vi "Dashboard Main.vi"() -> ()   [LabVIEW 2013]
uses:
  <vilib>/event_ctls.llb/eventvkey.ctl
  <vilib>/Rock Robotics/WPI/Dashboard/WPI_DashboardLogging Global.vi
  <vilib>/Utility/config.llb/Write Key (String).vi
  <vilib>/Utility/config.llb/Write Key (I32).vi
  <vilib>/Utility/config.llb/NI_LVConfig.lvlib
panel:
  out "LED 1":bool
  out "MotorSlide4 2":dbl(slide) scale=0.0..14.0 scale format="%#_2e"
  out "MotorSlide2 2":dbl(slide) scale=-1.0..1.0 scale format="%#_2e"
  out "MotorSlide1 2":dbl(slide) scale=-1.0..1.0 scale format="%#_2e"
  out "MotorSlide2":dbl(slide) scale=-1.0..1.0 scale format="%#_2e"
  out "MotorSlide1":dbl(slide) scale=-1.0..1.0 scale format="%#_2e"
  out "JS1 Z":dbl(slide) scale=-1.0..1.0 scale format="%#_2e"
  out "Joystick 1":cluster{"X":dbl, "Y":dbl}[](graph)
  out "JS Buttons 1":T1
  out "JS2 Z":dbl(slide) scale=-1.0..1.0 scale format="%#_2e"
  out "Joystick 2":cluster{"X":dbl, "Y":dbl}[](graph)
  out "JS Buttons 2":T1
  out "MotorChart R":cluster{"Numeric":dbl, "Numeric":dbl}(graph)
  out "MotorChart L":T2(graph)
  in  "DB Camera Config":bool
  out "fps":dbl format="%#.1g"
  out "Mbps":dbl format="%#.1g"
  out "Mbps 2":bool
  out "Image Message":string="Timeout in Camera Communications"
  in  "Rec Mode":enum32{"Stop", "Record", "Playback"}(radio)
  in  "Dashboard Tab":T3(tab)
  out "Posicionado?":bool
  out "Distância":dbl(slide)=60.0 scale=0.0..140.0 scale format="%#.3g"
  out "MARCHA":string
  out "Tração Invertida":bool
  out "Bola Coletada?":bool
  out "Engatilhado?":bool
  out "Claw Open?":bool
  out "Arm Down?":bool
  out "Shooter angle ready?":bool
  in  "Camera Settings":T4={"Frame Rate"=30, "Compression"=30, "Size"=1} {"Frame Rate" scale=1.0..30.0; "Size" items=["640x480", "320x240", "160x120"]}
  out "Mode":T5(ring)=enum."Auto Disabled"
  out "Camera IP":string
  in  "Checkbox 2":bool
  in  "Checkbox 1":bool
  in  "Test Slider":dbl(slide) scale=0.0..100.0 scale format="%#_3g"
  in  "On/Off":bool caption="Solenoid"
  in  "Test Name":u16(ring) items=["Select the test to run...", "Example Test", "-------------------------------", "List of tests is built in robot code.", "Replace with your own automated tests."]
  in  "Test Tree":string(tree)
  in  "Motor":cluster{"Value":dbl, "Enable":bool} {"Value" scale=-1.0..1.0 scale format="%#_3g"}
  out "Progress":T6 {"Test Progress" scale=0.0..100.0}
  in  "Rev/Fwd":cluster{"Forward":bool, "Reverse":bool}
  in  "Test Ring":u16(ring) items=["Auto", "Fixed indoor", "Fixed outdoor 1", "Fixed outdoor 2", "Fixed fluorescent 1", "Fixed fluorescent 2", "Hold current"]
  in  "Listbox":i32(listbox)
  out "Tree":string(tree)
  out "Camera Image":T7(plugin-control)
  in  "Enable":bool
  # "ABRIR\nGARRA"
  # "PARA"
  # "REVERTE"
  # "INTAKE"
  # "BRAÇO"
  # "SHOOT GOAL"
  # "SOLTA\nSHOOTER"
  # "SHOOT\nTRUSS"
  # "Left"
  # "Right"
  # "Front"
  # "Battery"
  # "Movimento Da Garra"
  # "Ações Da Garra"
  # "Tração"
  # "This tab is a great place for autonomous settings and validation.\nCustomize by placing controls and indicators here and name to\nmatch Dashboard Variables on robot."
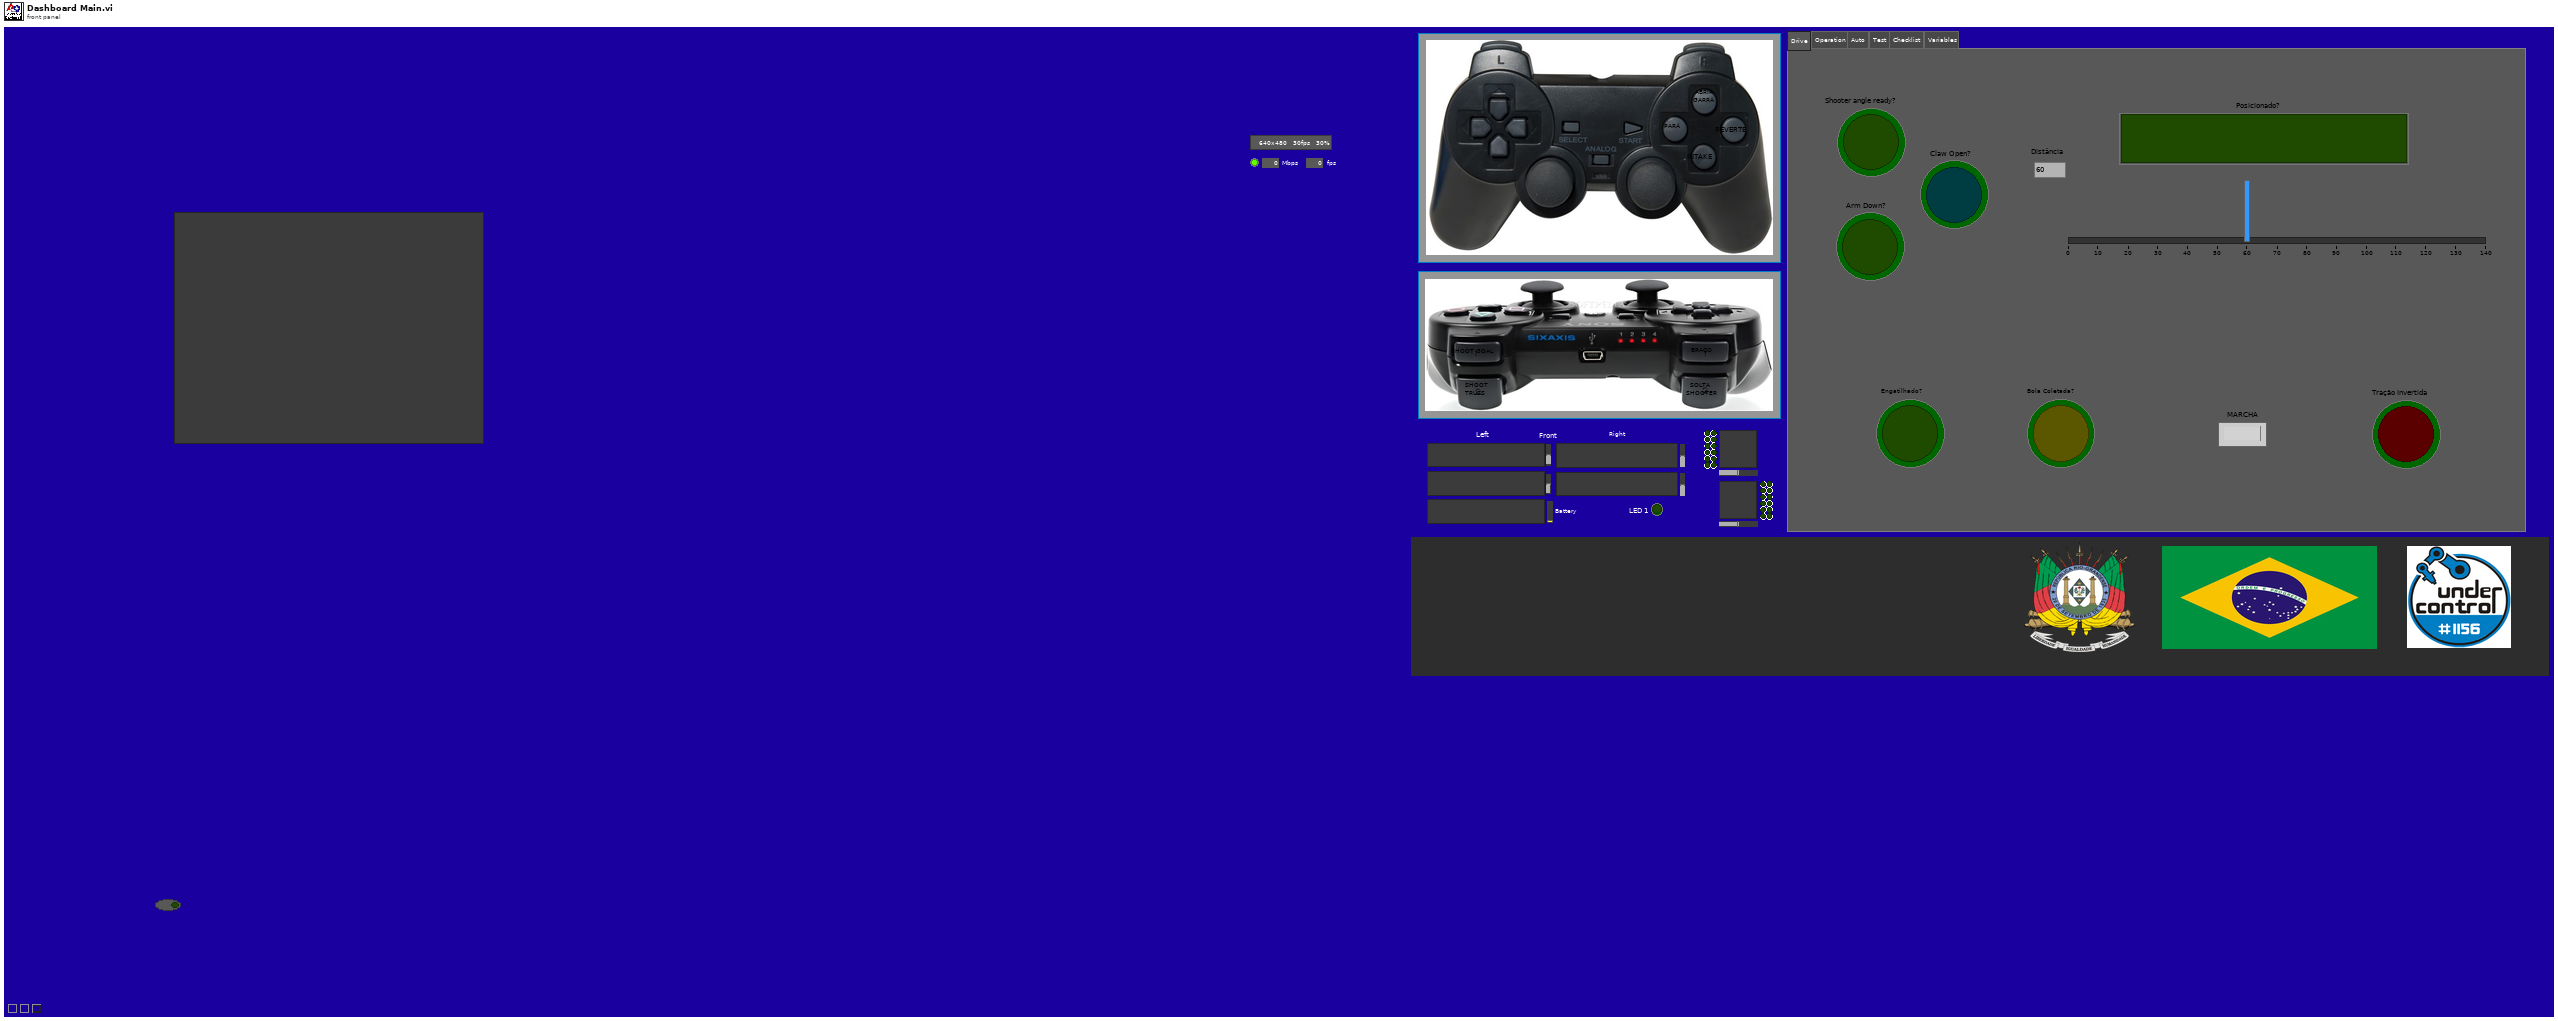
[diagram p1: front panel]
types:
  T1 = cluster{bool, bool, bool, bool, bool, bool, bool, bool, bool, bool, bool, bool}
  T2 = cluster{"Numeric":dbl, "Numeric":dbl, "Battery":sgl}
  T3 = enum32{"Drive", "Operation", "Auto", "Test", "Checklist", "Variables"}
  T4 = cluster{"Frame Rate":i32, "Compression":i32, "Size":u16}
  T5 = enum8{"Tele-Op Disabled", "Tele-Op Enabled", "Auto Disabled", "Auto Enabled", "Test Disabled", "Test Enabled", ""}
  T6 = cluster{"Test Progress":u8, "Test Progress Text":string}
  T7 = typedef "IMAQ Image.ctl" = refnum<image>
  T8 = typedef "Image Type" = u32
  T9 = cluster{"Digital Inputs":bool[], "Digital Outputs":bool[]}
  T10 = cluster{"Competition mode":bool, "Robot Link":bool, "Autonomous":bool, "Enabled":bool, "E-Stop":bool, "Simulated":bool, "TestMode":bool, "Docked Window":bool}
  T11 = cluster{"Boolean Array[0]":bool, "Boolean Array[1]":bool, "Boolean Array[2]":bool, "Boolean Array[3]":bool, "Boolean Array[4]":bool, "Boolean Array[5]":bool, "Boolean Array[6]":bool, "Boolean Array[7]":bool, "Boolean Array[8]":bool, "Boolean Array[9]":bool, "Boolean Array[10]":bool, "Boolean Array[11]":bool}
  T12 = typedef "NI_LVConfig.lvlib/Config Data RefNum.ctl" = refnum<k1>
  T13 = typedef "eventvkey.ctl" = enum16{"ASCII", "Enter", "Return", "Shift", "Ctrl", "Alt", "Cmd", "Opt", "Caps", "NumLock", "Clear", "Break", "Up", "Down", "Left", "Right", "Insert", "Delete", "Home", "End", "PageUp", "PageDown", "Escape", "Help", "Pause", "ScrollLock", "F1", "F2", "F3", "F4", "F5", "F6", "F7", "F8", "F9", "F10", "F11", "F12", "F13", "F14", "F15", "F16", "F17", "F18", "F19", "F20", "F21", "F22", "F23", "F24", "Play", "VolumeUp", "VolumeDown", "Mute", "Two Byte Char"}
  T14 = cluster{"Image Size":bool, "Image Type":bool, "Pixel Value":bool, "ROI Information":bool, "Zoom Factor":bool}
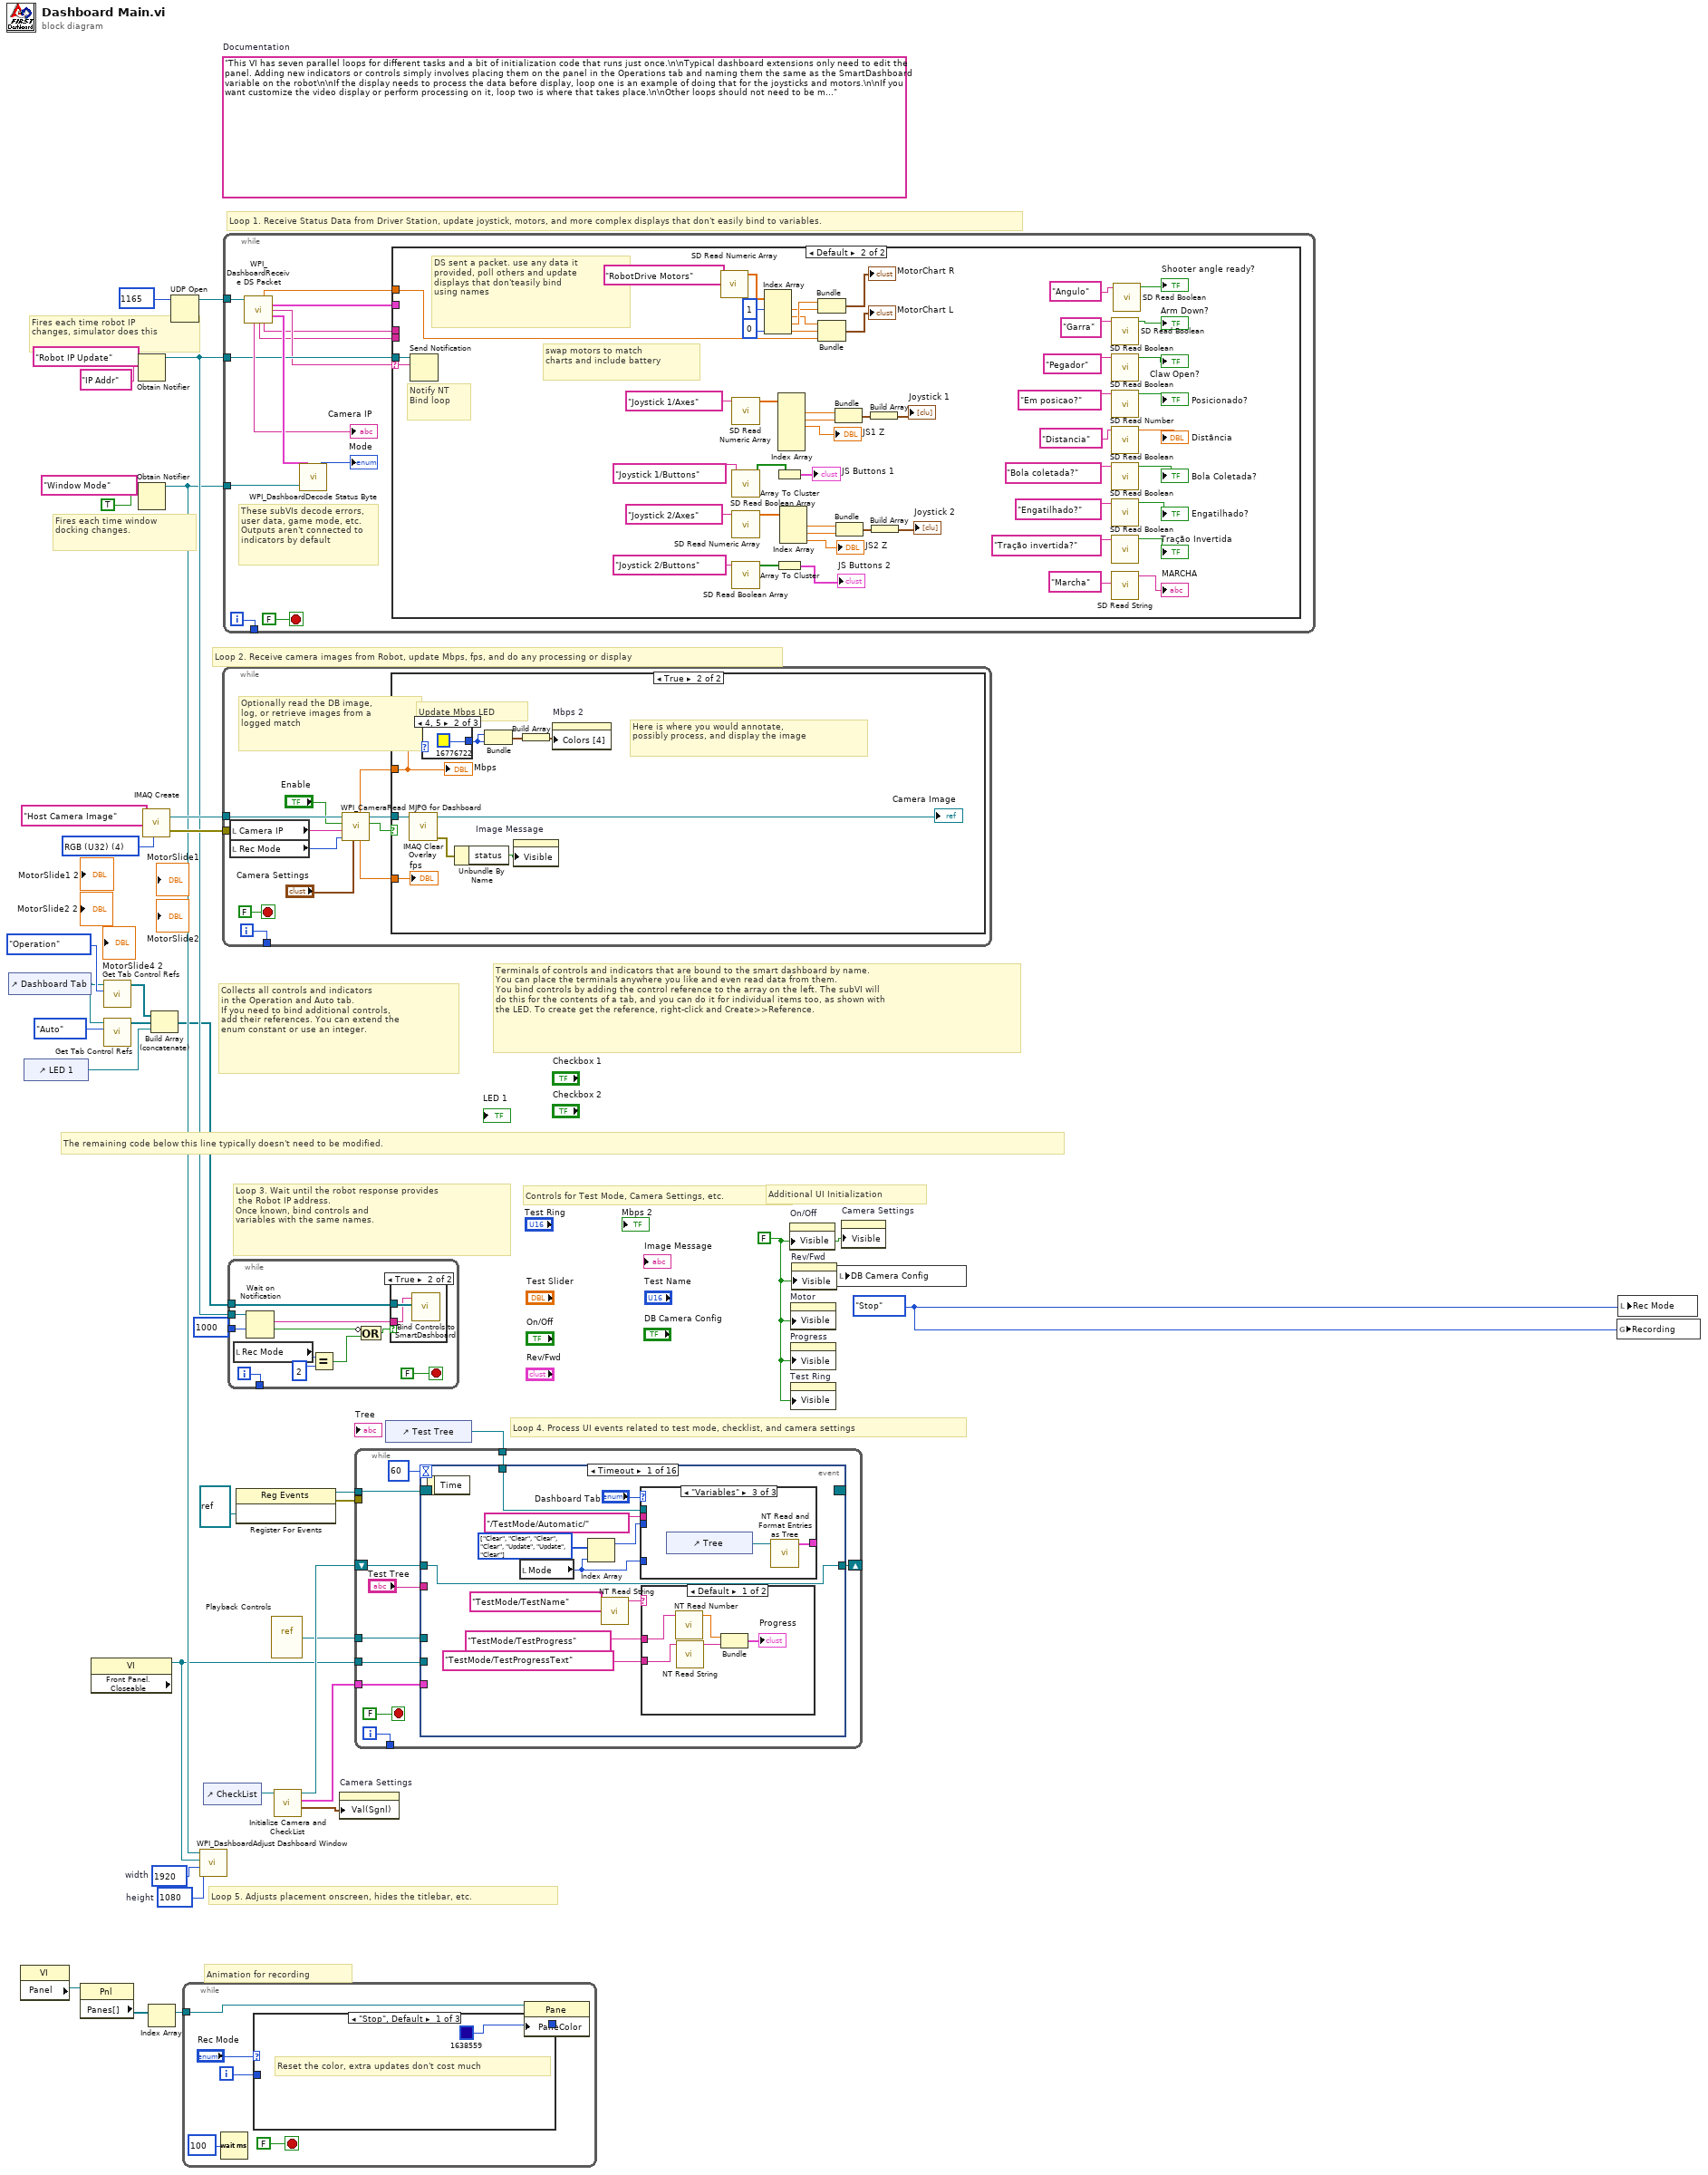
[diagram p0: block diagram]
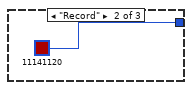
[diagram p2: hidden frame]
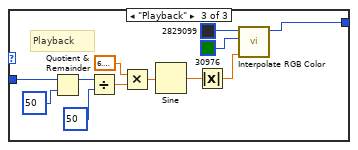
[diagram p3: hidden frame]
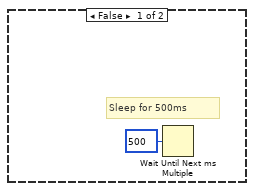
[diagram p5: hidden frame]
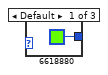
[diagram p6: hidden frame]
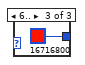
[diagram p7: hidden frame]
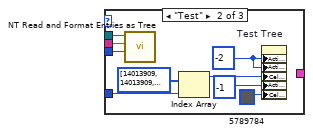
[diagram p9: hidden frame]
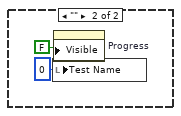
[diagram p10: hidden frame]
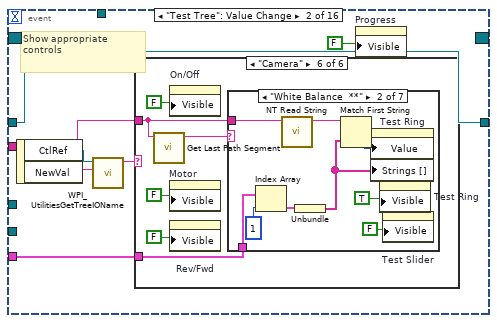
[diagram p11: hidden frame]
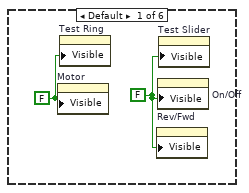
[diagram p12: hidden frame]
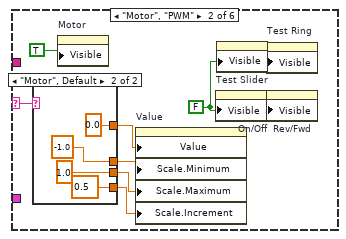
[diagram p13: hidden frame]
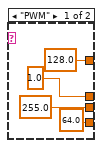
[diagram p14: hidden frame]
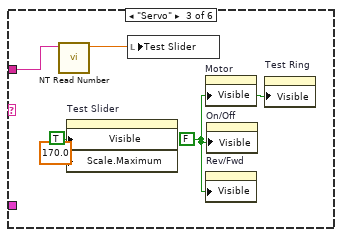
[diagram p15: hidden frame]
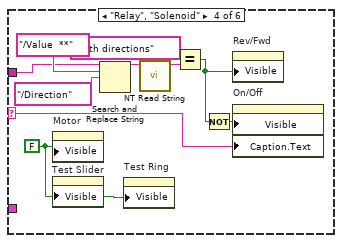
[diagram p16: hidden frame]
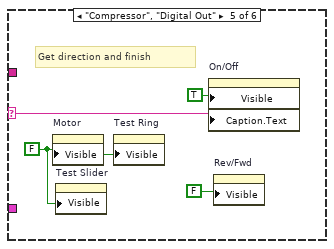
[diagram p17: hidden frame]
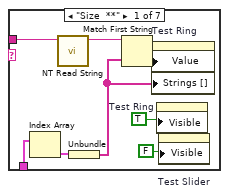
[diagram p18: hidden frame]
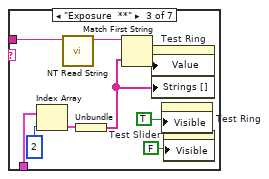
[diagram p19: hidden frame]
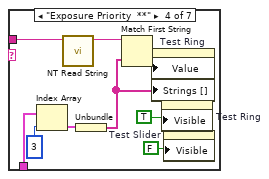
[diagram p20: hidden frame]
diagram:
  w8 = enum32{"Stop", "Record", "Playback"}."Stop" ("Rec Mode")
  w11 = 1080  # height
  w12 = 1920  # width
  w25 = FALSE ("Visible")
  (unwired) "This VI has seven parallel loops for different tasks and a bit of initialization code that runs just once.\n\nTypical dashboard extensions only need to edit the panel. Adding new indicators or controls simply involves placing them on the panel in the Operations tab and naming them the same as the SmartDashboard variable on the robot\n\nIf the display needs to process the data before display, loop one is an example of doing that for the joysticks and motors.\n\nIf you want customize the video display or perform processing on it, loop two is where that takes place.\n\nOther loops should not need to be modified. They are pretty standard, and document the task they perform."  # Documentation
  w35 = T8 4 items=["Grayscale (U8)", "Grayscale (I16)", "Grayscale (SGL)", "Complex (CSG)", "RGB (U32)", "HSL (U32)", "RGB (U64)"] ("Image Type")
  # "Controls for Test Mode, Camera Settings, etc."
  # "Additional UI Initialization"
  # "Animation for recording"
  # "Fires each time robot IP\nchanges, simulator does this"
  # "Fires each time window\ndocking changes."
  # "Collects all controls and indicators\nin the Operation and Auto tab.\nIf you need to bind additional controls,\nadd their references. You can extend the\nenum constant or use an integer."
  # "The remaining code below this line typically doesn't need to be modified."
  # "Loop 4. Process UI events related to test mode, checklist, and camera settings"
  # "Terminals of controls and indicators that are bound to the smart dashboard by name.\nYou can place the terminals anywhere you like and even read data from them.\nYou bind controls by adding the control reference to the array on the left. The subVI will\ndo this for the contents of a tab, and you can do it for individual items too, as shown with\nthe LED. To create get the reference, right-click and Create>>Reference."
  # "Loop 3. Wait until the robot response provides\n the Robot IP address.\nOnce known, bind controls and\nvariables with the same names."
  # "Loop 5. Adjusts placement onscreen, hides the titlebar, etc."
  # "Loop 1. Receive Status Data from Driver Station, update joystick, motors, and more complex displays that don't easily bind to variables."
  # "Loop 2. Receive camera images from Robot, update Mbps, fps, and do any processing or display"
  n1 = control-ref of="Dashboard Tab"() -> (w6:refnum<vi>)
  n2 = property class="VI"() -> ("Panel"=w19:refnum<vi>)  [unwired: 2 in, 2 out]
  n3 = control-ref of="LED 1"() -> (w1:refnum<vi>)
  n4 = property class="Pnl"(reference=w19) -> ("Panes[]"=w20:refnum<vi>[])  [unwired: 1 in, 2 out]
  n5 = property class="VI" props=["Front Panel.Closeable"]() -> (reference out=w7:refnum<vi>)  [unwired: 2 in, 2 out]
  n6 = call <vilib>:"Get Tab Control Refs.vi"("Page Index"=T3."Operation" ("Dashboard Tab"), "TabControl in"=w6) -> ("ControlsOnPage"=w4:refnum<vi>[])  [unwired: 9 in]
  n7 = call <vilib>:"Get Tab Control Refs.vi"("Page Index"=T3."Auto" ("Dashboard Tab"), "TabControl in"=w6) -> ("ControlsOnPage"=w5:refnum<vi>[])  [unwired: 9 in]
  n8 = Obtain Notifier(name (unnamed)="Robot IP Update", notification data type="IP Addr" ("name (unnamed)")) -> (notifier out=w29:refnum<notifier>)  [unwired: 2 in, 2 out]
  n9 = Obtain Notifier(name (unnamed)="Window Mode", notification data type=TRUE) -> (notifier out=w10:refnum<notifier>)  [unwired: 2 in, 2 out]
  n10 = call "IMAQ Create"("Image Name"="Host Camera Image", "Image Type"=w35) -> ("New Image"=w33:T7, "error out"=w32:errorcluster)  [unwired: 2 in, 1 out]
  n11 = Index Array(array=w20) -> (element=w18:refnum<vi>)  [unwired: 1 in]
  n12 = Build Array (concatenate)(w4, w5, w1) -> (w3:refnum<vi>[])
  n13 = UDP Open(11:u16 1165 ("port")) -> (port=w36:refnum<k16>)  [unwired: 2 in, 4 out]
  n14 = while {
    tunnel: w18 -> [w39]
    i -> [w42]
    stop <- FALSE stop-if-true
    n15 = Wait (ms)(milliseconds to wait=u32 100) -> ()  [unwired: 1 out]
    n16 = case shown="\"Stop\", Default" "Rec Mode" {
      tunnel: w42 -> [_ _ w57]
      tunnel: [u32 1638559 ("Base Color") u32 11141120 ("Target Color") w46] -> w38
      frame "Stop", Default {
        # "Reset the color, extra updates don't cost much"
      }
      frame "Record" {
      }
      frame "Playback" {
        # "Playback"
        n17 = Quotient & Remainder(x=w57, y=u32 50 ("milliseconds to wait")) -> (x-y*floor(x/y)=w53:u32)  [unwired: 1 out]
        n18 = Divide(x=w53, y=u32 50 ("milliseconds to wait")) -> (x/y=w50:dbl)
        n19 = Multiply(x=6.283185307179586, y=w50) -> (x*y=w55:dbl)
        n20 = Sine(x=w55) -> (sin(x)=w54:dbl)
        n21 = Absolute Value(x=w54) -> (abs(x)=w47:dbl)
        n22 = call "Interpolate RGB Color.vi"("Proportion"=w47, "Target Color"=u32 30976, "Base Color"=u32 2829099) -> ("Result Color"=w46:u32)  [unwired: 8 in]
      }
    }
    n23 = property class="Pane"(reference=w39, "PaneColor"=w38) -> ()  [unwired: 1 in, 2 out]
  }
  n24 = call <vilib>:"WPI_DashboardAdjust Dashboard Window.vi"("height"=w11, "width"=w12, "reference in"=w7, "Notifier in"=w10) -> ()  [unwired: 8 in]
  n25 = control-ref of="CheckList"() -> (w9:refnum<vi>)
  n26 = while {
    tunnel: w33 -> [w66]
    tunnel: w32 -> [_]
    tunnel: [w67] -> _
    i -> [w67]
    stop <- FALSE stop-if-true
    # "Optionally read the DB image,\nlog, or retrieve images from a\nlogged match"
    n27 = local read "Camera IP"() -> (w59:string)
    n28 = local read "Rec Mode"() -> (w58:enum32{"Stop", "Record", "Playback"})
    n29 = call <vilib>:"WPI_CameraRead MJPG for Dashboard.vi"("Camera Settings"="Camera Settings", "Rec Mode"=w58, "Camera IP"=w59, "Enable"="Enable", "Refnum in"=w66) -> ("Active"=w63:bool, "Refnum out"=w65:T7, "FPS"=w62:dbl, "Bandwidth (Mbps)"=w61:dbl)  [unwired: 3 in]
    n30 = case shown="True" w63 {
      tunnel: w65 -> [_ w73]
      tunnel: w61 -> [_ w72]
      tunnel: w62 -> [_ w70]
      frame False {
        # "Sleep for 500ms"
        n31 = Wait Until Next ms Multiple(millisecond multiple=u32 500) -> ()  [unwired: 1 out]
      }
      frame True {
        # "Here is where you would annotate,\npossibly process, and display the image"
        # "Update Mbps LED"
        n32 = call "IMAQ Clear Overlay"("Image"=w73) -> ("error out"=w77:errorcluster, "Image Out"=→"Camera Image":T7)  [unwired: 2 in, 7 out]
        n33 = case shown="4, 5" w72 {
          tunnel: [u32 6618880 ("Color Box") u32 16776722 ("Color Box") u32 16716800 ("Color Box")] -> w74
          frame Default {
          }
          frame 4, 5 {
          }
          frame 6.. {
          }
        }
        n34 = Unbundle By Name(w77) -> ("status"=w78:bool)
        n35 = Bundle("Color Box"=w74, "Color Box"=w74) -> (w76:cluster{"Color Box":u32, "Color Box":u32})  [unwired: 1 out]
        n36 = property on="Image Message" class="Str"("Visible"=w78) -> ()  [unwired: 2 in, 2 out]
        n37 = Build Array(w76) -> (w75:cluster{"Color Box":u32, "Color Box":u32}[])
        n38 = property on="Mbps 2" class="Bool (strict)"("Colors [4]"=w75) -> ()  [unwired: 2 in, 2 out]
        "Mbps" <- w72
        "fps" <- w70
      }
    }
  }
  n39 = while {
    tunnel: w36 -> [w92]
    tunnel: w29 -> [w87]
    tunnel: w10 -> [w91]
    tunnel: [w88] -> _
    i -> [w88]
    stop <- FALSE stop-if-true
    # "These subVIs decode errors, user data, game mode, etc.\nOutputs aren't connected to indicators by default"
    n40 = call <vilib>:"WPI_DashboardReceive DS Packet.vi"("Recv Socket"=w92) -> ("Battery"=w82:sgl, "Driver Station"=w83:T9, "Robot IP Address"=w86:string, "Status"=w93:T10, "Camera IP Address"=→"Camera IP":string, "Low Priority User Data"=w85:string, "High Priority User Data"=w84:string)  [unwired: 1 in, 7 out]
    n41 = call <vilib>:"WPI_DashboardDecode Status Byte.vi"("Window Mode Notifier"=w91, "Status"=w93) -> ("Mode"=→"Mode":T5)  [unwired: 1 out]
    n42 = case shown="Default" w86 {
      selector: w86 -> [_ w123]
      tunnel: w87 -> [_ w124]
      tunnel: w85 -> [_ _]
      tunnel: w84 -> [_ _]
      tunnel: w83 -> [_ _]
      tunnel: w82 -> [_ w122]
      frame "0.0.0.0" {
        # "DS not sending packets, or no robot exists yet.\nDon't poll the variables"
      }
      frame Default {
        # "Notify NT\nBind loop"
        # "DS sent a packet. use any data it\nprovided, poll others and update\ndisplays that don'teasily bind\nusing names"
        # "swap motors to match\ncharts and include battery"
        n43 = Send Notification(notification=w123, notifier=w124) -> ()  [unwired: 1 in, 2 out]
        n44 = call <vilib>:"SD Read Numeric Array.vi"("Name"="RobotDrive Motors") -> ("Numeric Array"=w121:dbl[])  [unwired: 8 in, 2 out]
        n45 = call <vilib>:"SD Read Numeric Array.vi"("Name"="Joystick 1/Axes") -> ("Numeric Array"=w140:dbl[])  [unwired: 8 in, 2 out]
        n46 = call <vilib>:"SD Read Boolean Array.vi"("Name"="Joystick 1/Buttons") -> ("Boolean Array"=w142:bool[])  [unwired: 8 in, 2 out]
        n47 = call <vilib>:"SD Read Numeric Array.vi"("Name"="Joystick 2/Axes") -> ("Numeric Array"=w134:dbl[])  [unwired: 8 in, 2 out]
        n48 = call <vilib>:"SD Read Boolean Array.vi"("Name"="Joystick 2/Buttons") -> ("Boolean Array"=w133:bool[])  [unwired: 8 in, 2 out]
        n49 = Index Array(array=w121, index #1=1, index #4=0) -> (element #1=w119:dbl, element #2=w118:dbl, element #3=w120:dbl, element #4=w115:dbl)  [unwired: 2 in]
        n50 = Array To Cluster(array=w142) -> (cluster=→"JS Buttons 1":T11)
        n51 = Array To Cluster(array=w133) -> (cluster=→"JS Buttons 2":T11)
        n52 = Index Array(array=w140) -> (element #1=w137:dbl, element #2=w138:dbl, element #3=→"JS1 Z":dbl)  [unwired: 6 in, 3 out]
        n53 = Index Array(array=w134) -> (element #1=w129:dbl, element #2=w128:dbl, element #3=→"JS2 Z":dbl)  [unwired: 3 in]
        n54 = Bundle("Numeric"=w120, "Numeric"=w119) -> (→"MotorChart R":cluster{"Numeric":dbl, "Numeric":dbl})  [unwired: 1 in]
        n55 = Bundle("Numeric"=w118, "Numeric"=w115, "Battery"=w122) -> (→"MotorChart L":T2)  [unwired: 1 in]
        n56 = Bundle("Numeric"=w137, "Numeric"=w138) -> (w136:cluster{"Numeric":dbl, "Numeric":dbl})  [unwired: 1 in]
        n57 = Bundle("Numeric"=w129, "Numeric"=w128) -> (w130:cluster{"Numeric":dbl, "Numeric":dbl})  [unwired: 1 in]
        n58 = Build Array(w136) -> (→"Joystick 1":cluster{"Numeric":dbl, "Numeric":dbl}[])
        n59 = Build Array(w130) -> (→"Joystick 2":cluster{"Numeric":dbl, "Numeric":dbl}[])
        n60 = call <vilib>:"SD Read Boolean.vi"("Name"="Garra") -> ("Boolean"=→"Arm Down?":bool)  [unwired: 8 in, 2 out]
        n61 = call <vilib>:"SD Read Boolean.vi"("Name"="Pegador") -> ("Boolean"=→"Claw Open?":bool)  [unwired: 8 in, 2 out]
        n62 = call <vilib>:"SD Read Boolean.vi"("Name"="Em posicao?") -> ("Boolean"=→"Posicionado?":bool)  [unwired: 8 in, 2 out]
        n63 = call <vilib>:"SD Read Number.vi"("Name"="Distancia") -> ("Numeric"=→"Distância":dbl)  [unwired: 8 in, 2 out]
        n64 = call <vilib>:"SD Read Boolean.vi"("Name"="Bola coletada?") -> ("Boolean"=→"Bola Coletada?":bool)  [unwired: 8 in, 2 out]
        n65 = call <vilib>:"SD Read Boolean.vi"("Name"="Engatilhado?") -> ("Boolean"=→"Engatilhado?":bool)  [unwired: 8 in, 2 out]
        n66 = call <vilib>:"SD Read Boolean.vi"("Name"="Tração invertida?") -> ("Boolean"=→"Tração Invertida":bool)  [unwired: 8 in, 2 out]
        n67 = call <vilib>:"SD Read String.vi"("Name"="Marcha") -> ("String"=→"MARCHA":string)  [unwired: 8 in, 2 out]
        n68 = call <vilib>:"SD Read Boolean.vi"("Name"="Angulo") -> ("Boolean"=→"Shooter angle ready?":bool)  [unwired: 8 in, 2 out]
      }
    }
  }
  n69 = while {
    tunnel: w3 -> [w156]
    tunnel: w29 -> [w154]
    tunnel: [w152] -> _
    tunnel: u32 1000 ("milliseconds to wait") -> [w151]
    i -> [w152]
    stop <- FALSE stop-if-true
    n70 = local read "Rec Mode"() -> (w147:enum32{"Stop", "Record", "Playback"})
    n71 = Wait on Notification(notifier=w154, timeout in ms (-1)=w151) -> (notification=w153:string, timed out?=w149:bool)  [unwired: 2 in, 2 out]
    n72 = Equal?(x=w147, y=u16 2 ("Rec Mode")) -> (x = y?=w148:bool)
    n73 = Compound Arithmetic op=OR(invert w149, w148) -> (w150:bool)
    n74 = case shown="True" w150 {
      tunnel: w156 -> [_ w158]
      tunnel: w153 -> [_ w157]
      frame False {
      }
      frame True {
        n75 = call <vilib>:"Bind Controls to SmartDashboard.vi"("Bound Control Refs"=w158, "Server IP Address"=w157) -> ()  [unwired: 10 in]
      }
    }
  }
  n76 = register-events(refnum<vi> refnum) -> (reference out=w16:refnum<event-registration>, error out=w15:errorcluster)  [unwired: 2 in]
  n77 = vi-ref "Playback Controls.vi"() -> (w17:refnum<vi>)
  n78 = call "Initialize Camera and CheckList.vi"("ListBox in"=w9) -> ("Cluster"=w23:cluster{"value":i32, "value":i32, "index":i32}, "Array"=w24:cluster{string[]}[], "File Refnum"=w22:T12)  [unwired: 8 in]
  n79 = property on="Camera Settings" class="Clust (strict)"("Val(Sgnl)"=w23) -> ()  [unwired: 2 in, 2 out]
  n80 = control-ref of="Test Tree"() -> (w21:refnum<vi>)
  n81 = while {
    tunnel: w24 -> [w166]
    shift-right: [w165] -> _
    shift-left: w22 -> [w164]
    tunnel: [w163] -> _
    tunnel: w21 -> [w162]
    tunnel: w17 -> [w161]
    tunnel: w16 -> [w160]
    tunnel: w15 -> [_]
    tunnel: w7 -> [w159]
    i -> [w163]
    stop <- FALSE stop-if-true
    n82 = event shown="[0] Timeout" {
      selector: w160 -> [_ _ _ _ _ _ _ _ _ _ _ _ _ _ _ _]
      dyn-events: [_ _ _ _ _ _ _ _ _ _ _ _ _ w404 _ _] -> _
      timeout: u32 60 ("milliseconds to wait") -> [_ _ _ _ _ _ _ _ _ _ _ _ _ _ _ _]
      tunnel: w162 -> [w176 _ _ _ _ _ _ _ _ _ _ _ _ _ _ _]
      tunnel: "Test Tree" -> [_ _ _ _ _ _ _ _ w373 w381 w383 w387 w395 _ _ _]
      tunnel: w166 -> [_ w200 _ _ _ _ w337 w367 _ _ _ _ _ _ _ _]
      tunnel: [w170 w199 w298 w303 w311 w323 w336 w360 w372 w379 w382 w386 w394 w406 w420 w421] -> w165
      tunnel: w164 -> [w170 w199 w298 w303 w311 w323 w335 w360 w372 w379 w382 w386 w394 w406 w420 w421]
      tunnel: w161 -> [_ _ _ _ _ _ _ _ _ _ _ _ _ w407 _ w424]
      tunnel: w159 -> [_ _ _ _ _ _ _ _ _ _ _ _ _ w402 _ _]
      event Timeout {
        w175 = enum16{"Update", "Clear"}[] [enum."Clear", enum."Clear", enum."Clear", enum."Clear", enum."Update", enum."Update", enum."Clear"] items=["Update", "Clear"]
        n83 = event-data() -> ()  [unwired: 1 in, 1 out]
        n84 = local read "Mode"() -> (w173:T5)
        n85 = Index Array(array=w175, index=w173) -> (element=w174:enum16{"Update", "Clear"})
        n86 = call <vilib>:"NT Read String.vi"("Name"="TestMode/TestName") -> ("String"=w179:string)  [unwired: 9 in, 1 out]
        n87 = case shown="\"Variables\"" "Dashboard Tab" {
          tunnel: w176 -> [_ w189 _]
          tunnel: "/TestMode/Automatic/" ("Name Pattern") -> [_ w188 _]
          tunnel: w174 -> [_ w187 _]
          tunnel: w173 -> [_ w185 _]
          tunnel: [_ _ w191] -> _
          frame "Operation", Default {
          }
          frame "Test" {
            w184 = -2 ("Active Item:Row Number")
            n88 = call <vilib>:"NT Read and Format Entries as Tree.vi"("Operation"=w187, "Name Pattern"=w188, "Tree Refnum"=w189) -> ()  [unwired: 7 in, 2 out]
            n89 = Index Array(array=u32[] [14013909, 14013909, 14013909, 14013909, 14013909, 16777215, 14013909], index=w185) -> (element=w183:u32)
            n90 = property on="Test Tree" class="Tree (strict)"("Active Item Row Number"=w184, "ActiveColNum"=w184, "CellBG"=w183, "Active Item Row Number"=-1 ("Active Item:Row Number"), "CellBG"=u32 5789784 ("Color Box")) -> ()  [unwired: 2 in, 2 out]
          }
          frame "Variables" {
            n91 = control-ref of="Tree"() -> (w190:refnum<vi>)
            n92 = call <vilib>:"NT Read and Format Entries as Tree.vi"("Tree Refnum"=w190) -> ("Formatted Strings"=w191:cluster{"Name":string, "Value":string}[])  [unwired: 9 in, 1 out]
          }
        }
        n93 = case shown="Default" w179 {
          tunnel: "TestMode/TestProgress" ("Name") -> [w193 _]
          tunnel: "TestMode/TestProgressText" ("Name") -> [w192 _]
          frame Default {
            n94 = call <vilib>:"NT Read Number.vi"("Name"=w193) -> ("Numeric"=w194:dbl)  [unwired: 9 in, 1 out]
            n95 = call <vilib>:"NT Read String.vi"("Name"=w192) -> ("String"=w195:string)  [unwired: 9 in, 1 out]
            n96 = Bundle("Numeric"=w194, "String"=w195) -> (→"Progress":cluster{"Numeric":dbl, "String":string})  [unwired: 1 in]
          }
          frame "" {
            n97 = local write "Test Name"(u16 0) -> ()
            n98 = property on="Progress" class="Clust (strict)"("Visible"=FALSE) -> ()  [unwired: 2 in, 2 out]
          }
        }
      }
      event "Test Tree": Value Change {
        # "Show appropriate\ncontrols"
        n99 = event-data() -> ("CtlRef"=w203:refnum<vi>, "NewVal"=w201:string)  [unwired: 1 in]
        n100 = call <vilib>:"WPI_UtilitiesGetTreeIOName.vi"("NewVal"=w201, "TreeControl in"=w203) -> ("I/O Name"=w204:string)  [unwired: 9 in]
        n101 = case shown="\"Camera\"" w204 {
          selector: w204 -> [_ w211 _ w229 w238 _]
          tunnel: w201 -> [_ _ w226 w228 _ w245]
          tunnel: w200 -> [_ _ _ _ _ w244]
          frame Default {
            w206 = FALSE ("Visible")
            w205 = FALSE ("Visible")
            n102 = property on="Motor" class="Clust (strict)"("Visible"=w205) -> ()  [unwired: 2 in, 2 out]
            n103 = property on="Test Ring" class="Ring (strict)"("Visible"=w205) -> ()  [unwired: 2 in, 2 out]
            n104 = property on="Rev/Fwd" class="Clust (strict)"("Visible"=w206) -> ()  [unwired: 2 in, 2 out]
            n105 = property on="On/Off" class="Bool (strict)"("Visible"=w206) -> ()  [unwired: 2 in, 2 out]
            n106 = property on="Test Slider" class="Slide (strict)"("Visible"=w206) -> ()  [unwired: 2 in, 2 out]
          }
          frame "Motor", "PWM" {
            w212 = FALSE ("Visible")
            n107 = case shown="\"Motor\", Default" w211 {
              tunnel: [1.0 ("Value") -1.0 ("Value")] -> w210
              tunnel: [255.0 ("Value") 1.0 ("Value")] -> w209
              tunnel: [128.0 ("Value") 0.0 ("Value")] -> w208
              tunnel: [64.0 ("Value") 0.5 ("Value")] -> w207
              frame "PWM" {
              }
              frame "Motor", Default {
              }
            }
            n108 = property on="Motor" class="Clust (strict)"("Visible"=TRUE) -> ()  [unwired: 2 in, 2 out]
            n109 = property on="Value" class="Slide (strict)"("Value"=w208, "Scale.Minimum"=w210, "Scale.Maximum"=w209, "Scale.Increment"=w207) -> ()  [unwired: 2 in, 2 out]
            n110 = property on="On/Off" class="Bool (strict)"("Visible"=w212) -> ()  [unwired: 2 in, 2 out]
            n111 = property on="Test Slider" class="Slide (strict)"("Visible"=w212) -> ()  [unwired: 2 in, 2 out]
            n112 = property on="Test Ring" class="Ring (strict)"("Visible"=w212) -> ()  [unwired: 2 in, 2 out]
            n113 = property on="Rev/Fwd" class="Clust (strict)"("Visible"=w212) -> ()  [unwired: 2 in, 2 out]
          }
          frame "Servo" {
            w224 = FALSE ("Visible")
            n114 = call <vilib>:"NT Read Number.vi"("Name"=w226) -> ("Numeric"=w225:dbl)  [unwired: 9 in, 1 out]
            n115 = property on="Test Slider" class="Slide (strict)"("Visible"=TRUE, "Scale.Maximum"=170.0 ("Scale.Range:Maximum")) -> ()  [unwired: 2 in, 2 out]
            n116 = local write "Test Slider"(w225) -> ()
            n117 = property on="Motor" class="Clust (strict)"("Visible"=w224) -> ()  [unwired: 2 in, 2 out]
            n118 = property on="Rev/Fwd" class="Clust (strict)"("Visible"=w224) -> ()  [unwired: 2 in, 2 out]
            n119 = property on="On/Off" class="Bool (strict)"("Visible"=w224) -> ()  [unwired: 2 in, 2 out]
            n120 = property on="Test Ring" class="Ring (strict)"("Visible"=w224) -> ()  [unwired: 2 in, 2 out]
          }
          frame "Relay", "Solenoid" {
            w227 = FALSE ("Visible")
            n121 = property on="Motor" class="Clust (strict)"("Visible"=w227) -> ()  [unwired: 2 in, 2 out]
            n122 = property on="Test Slider" class="Slide (strict)"("Visible"=w227) -> ()  [unwired: 2 in, 2 out]
            n123 = Search and Replace String(input string=w228, search string="/Value  **", replace string="/Direction") -> (result string=w234:string)  [unwired: 5 in, 3 out]
            n124 = property on="Test Ring" class="Ring (strict)"("Visible"=w227) -> ()  [unwired: 2 in, 2 out]
            n125 = call <vilib>:"NT Read String.vi"("Name"=w234) -> ("String"=w232:string)  [unwired: 9 in, 1 out]
            n126 = Equal?(x="Both directions", y=w232) -> (x = y?=w230:bool)
            n127 = Not(x=w230) -> (.not. x?=w231:bool)
            n128 = property on="Rev/Fwd" class="Clust (strict)"("Visible"=w230) -> ()  [unwired: 2 in, 2 out]
            n129 = property on="On/Off" class="Bool (strict)"("Visible"=w231, "Caption.Text"=w229) -> ()  [unwired: 2 in, 2 out]
          }
          frame "Compressor", "Digital Out" {
            w237 = FALSE ("Visible")
            # "Get direction and finish"
            n130 = property on="Motor" class="Clust (strict)"("Visible"=w237) -> ()  [unwired: 2 in, 2 out]
            n131 = property on="Test Slider" class="Slide (strict)"("Visible"=w237) -> ()  [unwired: 2 in, 2 out]
            n132 = property on="Test Ring" class="Ring (strict)"("Visible"=w237) -> ()  [unwired: 2 in, 2 out]
            n133 = property on="On/Off" class="Bool (strict)"("Visible"=TRUE, "Caption.Text"=w238) -> ()  [unwired: 2 in, 2 out]
            n134 = property on="Rev/Fwd" class="Clust (strict)"("Visible"=FALSE) -> ()  [unwired: 2 in, 2 out]
          }
          frame "Camera" {
            n135 = call <vilib>:"Get Last Path Segment.vi"("String in"=w245) -> ("String out"=w246:string)  [unwired: 10 in]
            n136 = property on="On/Off" class="Bool (strict)"("Visible"=FALSE) -> ()  [unwired: 2 in, 2 out]
            n137 = property on="Motor" class="Clust (strict)"("Visible"=FALSE) -> ()  [unwired: 2 in, 2 out]
            n138 = property on="Rev/Fwd" class="Clust (strict)"("Visible"=FALSE) -> ()  [unwired: 2 in, 2 out]
            n139 = case shown="\"White Balance  **\"" w246 {
              tunnel: w245 -> [w252 w261 w270 w279 w288 _ w294]
              tunnel: w244 -> [w250 w258 w267 w276 w285 _ _]
              frame "Size  **" {
                n140 = Index Array(array=w250) -> (element=w249:cluster{string[]})  [unwired: 1 in]
                n141 = call <vilib>:"NT Read String.vi"("Name"=w252) -> ("String"=w251:string)  [unwired: 9 in, 1 out]
                n142 = Unbundle(w249) -> (w247:string[])
                n143 = Match First String(2:w247, 3:w251) -> (0:w248:i32)  [unwired: 1 out]
                n144 = property on="Test Ring" class="Ring (strict)"("Value"=w248, "Strings []"=w247) -> ()  [unwired: 2 in, 2 out]
                n145 = property on="Test Ring" class="Ring (strict)"("Visible"=TRUE) -> ()  [unwired: 2 in, 2 out]
                n146 = property on="Test Slider" class="Slide (strict)"("Visible"=FALSE) -> ()  [unwired: 2 in, 2 out]
              }
              frame "White Balance  **" {
                n147 = Index Array(array=w258, index=1) -> (element=w259:cluster{string[]})
                n148 = call <vilib>:"NT Read String.vi"("Name"=w261) -> ("String"=w260:string)  [unwired: 9 in, 1 out]
                n149 = Unbundle(w259) -> (w256:string[])
                n150 = Match First String(2:w256, 3:w260) -> (0:w255:i32)  [unwired: 1 out]
                n151 = property on="Test Ring" class="Ring (strict)"("Value"=w255, "Strings []"=w256) -> ()  [unwired: 2 in, 2 out]
                n152 = property on="Test Ring" class="Ring (strict)"("Visible"=TRUE) -> ()  [unwired: 2 in, 2 out]
                n153 = property on="Test Slider" class="Slide (strict)"("Visible"=FALSE) -> ()  [unwired: 2 in, 2 out]
              }
              frame "Exposure  **" {
                n154 = Index Array(array=w267, index=2) -> (element=w268:cluster{string[]})
                n155 = call <vilib>:"NT Read String.vi"("Name"=w270) -> ("String"=w269:string)  [unwired: 9 in, 1 out]
                n156 = Unbundle(w268) -> (w264:string[])
                n157 = Match First String(2:w264, 3:w269) -> (0:w265:i32)  [unwired: 1 out]
                n158 = property on="Test Ring" class="Ring (strict)"("Value"=w265, "Strings []"=w264) -> ()  [unwired: 2 in, 2 out]
                n159 = property on="Test Ring" class="Ring (strict)"("Visible"=TRUE) -> ()  [unwired: 2 in, 2 out]
                n160 = property on="Test Slider" class="Slide (strict)"("Visible"=FALSE) -> ()  [unwired: 2 in, 2 out]
              }
              frame "Exposure Priority  **" {
                n161 = Index Array(array=w276, index=3) -> (element=w277:cluster{string[]})
                n162 = call <vilib>:"NT Read String.vi"("Name"=w279) -> ("String"=w278:string)  [unwired: 9 in, 1 out]
                n163 = Unbundle(w277) -> (w273:string[])
                n164 = Match First String(2:w273, 3:w278) -> (0:w274:i32)  [unwired: 1 out]
                n165 = property on="Test Ring" class="Ring (strict)"("Value"=w274, "Strings []"=w273) -> ()  [unwired: 2 in, 2 out]
                n166 = property on="Test Ring" class="Ring (strict)"("Visible"=TRUE) -> ()  [unwired: 2 in, 2 out]
                n167 = property on="Test Slider" class="Slide (strict)"("Visible"=FALSE) -> ()  [unwired: 2 in, 2 out]
              }
              frame "Color Enable  **" {
                n168 = Index Array(array=w285, index=4) -> (element=w286:cluster{string[]})
                n169 = call <vilib>:"NT Read String.vi"("Name"=w288) -> ("String"=w287:string)  [unwired: 9 in, 1 out]
                n170 = Unbundle(w286) -> (w282:string[])
                n171 = Match First String(2:w282, 3:w287) -> (0:w283:i32)  [unwired: 1 out]
                n172 = property on="Test Ring" class="Ring (strict)"("Value"=w283, "Strings []"=w282) -> ()  [unwired: 2 in, 2 out]
                n173 = property on="Test Ring" class="Ring (strict)"("Visible"=TRUE) -> ()  [unwired: 2 in, 2 out]
                n174 = property on="Test Slider" class="Slide (strict)"("Visible"=FALSE) -> ()  [unwired: 2 in, 2 out]
              }
              frame Default {
                n175 = property on="Test Ring" class="Ring (strict)"("Visible"=FALSE) -> ()  [unwired: 2 in, 2 out]
                n176 = property on="Test Slider" class="Slide (strict)"("Visible"=FALSE) -> ()  [unwired: 2 in, 2 out]
              }
              frame "Brightness  **", "Color Level  **", "Compression  **", "FPS  **", "Sharpness  **" {
                n177 = call <vilib>:"NT Read Number.vi"("Name"=w294) -> ("Numeric"=w293:dbl)  [unwired: 9 in, 1 out]
                n178 = local write "Test Slider"(w293) -> ()
                n179 = property on="Test Slider" class="Slide (strict)"("Visible"=TRUE, "Scale.Maximum"=100.0 ("Scale.Range:Maximum")) -> ()  [unwired: 2 in, 2 out]
                n180 = property on="Test Ring" class="Ring (strict)"("Visible"=FALSE) -> ()  [unwired: 2 in, 2 out]
              }
            }
          }
        }
        n181 = property on="Progress" class="Clust (strict)"("Visible"=FALSE) -> ()  [unwired: 2 in, 2 out]
      }
      event "Test Name": Mouse Enter {
        # "Populate the ring with the list of tests"
        n182 = event-data() -> ()  [unwired: 1 in, 1 out]
        n183 = call <vilib>:"NT Read String Array.vi"("Name"="TestMode/TestList") -> ("String Array"=w302:string[])  [unwired: 9 in, 1 out]
        n184 = Build Array (concatenate)("Select the test to run...", w302) -> (w301:string[])
        n185 = property on="Test Name" class="Ring (strict)"("Strings []"=w301) -> ()  [unwired: 2 in, 2 out]
      }
      event "Test Name": Value Change {
        w304 = FALSE ("Visible")
        # "Tell the robot the test name to run"
        n186 = event-data() -> ("NewVal"=w308:u16)  [unwired: 1 in]
        n187 = property on="Test Name" class="Ring (strict)"() -> ("Strings []"=w309:string[])  [unwired: 2 in, 2 out]
        n188 = local write "Progress"(T6 {"Test Progress"=0, "Test Progress Text"=""} ("Progress")) -> ()
        n189 = Index Array(array=w309, index=w308) -> (element=w307:string)
        n190 = call <vilib>:"NT Write String.vi"("String"=w307, "Name"="TestMode/TestName") -> ()  [unwired: 9 in, 1 out]
        n191 = property on="Progress" class="Clust (strict)"("Visible"=TRUE) -> ()  [unwired: 2 in, 2 out]
        n192 = property on="Motor" class="Clust (strict)"("Visible"=w304) -> ()  [unwired: 2 in, 2 out]
        n193 = property on="Test Slider" class="Slide (strict)"("Visible"=w304) -> ()  [unwired: 2 in, 2 out]
        n194 = property on="On/Off" class="Bool (strict)"("Visible"=w304) -> ()  [unwired: 2 in, 2 out]
        n195 = property on="Rev/Fwd" class="Clust (strict)"("Visible"=w304) -> ()  [unwired: 2 in, 2 out]
        n196 = property on="Test Ring" class="Ring (strict)"("Visible"=w304) -> ()  [unwired: 2 in, 2 out]
      }
      event "Listbox": Double Click {
        n197 = event-data() -> ("PlatMods.Shift"=w312:bool, "Row"=w314:i32)  [unwired: 1 in]
        n198 = case shown="True" w312 {
          tunnel: w314 -> [w318 _]
          tunnel: 1 -> [w317 _]
          frame False {
            n199 = property on="Listbox" class="LstBox (strict)"() -> ("Item Symbols"=w316:i32[])  [unwired: 2 in, 2 out]
            n200 = Replace Array Subset(array=w316, new element=w317, index=w318) -> (w315:i32[])
            n201 = property on="Listbox" class="LstBox (strict)"("Item Symbols"=w315) -> ()  [unwired: 2 in, 2 out]
          }
          frame True {
            w319 = 0 ("Top Row")
            n202 = property on="Listbox" class="LstBox (strict)"() -> ("Number of Rows"=w321:u32)  [unwired: 2 in, 2 out]
            n203 = Initialize Array(0, w321) -> (w320:i32[])
            n204 = property on="Listbox" class="LstBox (strict)"("Top Row"=w319, "Value"=w319, "Item Symbols"=w320) -> ()  [unwired: 2 in, 2 out]
          }
        }
      }
      event "Listbox": Key Down {
        n205 = event-data() -> ("VKey"=w325:T13)  [unwired: 1 in]
        n206 = case shown="\"Left\", \"Right\"" w325 {
          selector: w325 -> [w330 _]
          tunnel: eventvkey."Left" ("VKey") -> [w328 _]
          frame "Left", "Right" {
            n207 = Equal?(x=w328, y=w330) -> (x = y?=w329:bool)
            n208 = Select(t=0, s=w329, f=1) -> (s? t:f=w331:i32)
            n209 = property on="Listbox" class="LstBox (strict)"() -> ("Item Symbols"=w334:i32[])  [unwired: 2 in, 2 out]
            n210 = Replace Array Subset(array=w334, new element=w331, index="Listbox") -> (w333:i32[])
            n211 = property on="Listbox" class="LstBox (strict)"("Item Symbols"=w333) -> ()  [unwired: 2 in, 2 out]
          }
          frame Default {
          }
        }
      }
      event "DB Camera Config": Value Change {
        n212 = event-data() -> ("NewVal"=w338:bool)  [unwired: 1 in]
        n213 = case shown="False" w338 {
          tunnel: w337 -> [w347 _]
          tunnel: [w340 w358] -> w336
          tunnel: w335 -> [w339 w358]
          frame False {
            w354 = "Camera"
            w357 = FALSE ("Visible")
            n214 = local read "Camera Settings"() -> (w346:T4)
            n215 = Index Array(array=w347) -> (element=w350:cluster{string[]})  [unwired: 1 in]
            n216 = Unbundle(w346) -> ("Frame Rate"=w345:i32, "Compression"=w344:i32, "Size"=w348:u16)
            n217 = Unbundle(w350) -> (w349:string[])
            n218 = Index Array(array=w349, index=w348) -> (element=w343:string)
            n219 = call-poly <vilib>:"Write Key.vi"("section"=w354, "value"=w343, "key"="Size", "refnum"=w339) -> ("refnum out"=w356:T12)  [unwired: 2 in, 5 out]
            n220 = call-poly <vilib>:"Write Key.vi"("section"=w354, "value"=w345, "key"="FrameRate", "refnum"=w356) -> ("refnum out"=w355:T12)  [unwired: 1 in, 6 out]
            n221 = local write "DB Camera Config"(w357) -> ()
            n222 = property on="Camera Settings" class="Clust (strict)"("Visible"=w357) -> ()  [unwired: 2 in, 2 out]
            n223 = call-poly <vilib>:"Write Key.vi"("section"=w354, "value"=w344, "key"="Compression", "refnum"=w355) -> ("refnum out"=w341:T12)  [unwired: 1 in, 6 out]
            n224 = call <vilib>:"Close Config Data.vi"("refnum"=w341) -> ("file path"=w342:path)  [unwired: 2 in, 8 out]
            n225 = call <vilib>:"Open Config Data.vi"("configuration file path"=w342) -> ("refnum"=w340:T12)  [unwired: 8 in, 2 out]
          }
          frame True {
            n226 = property on="Camera Settings" class="Clust (strict)"("Visible"=TRUE) -> ()  [unwired: 2 in, 2 out]
          }
        }
      }
      event "Camera Settings": Value Change {
        n227 = event-data() -> ("NewVal"=w371:T4)  [unwired: 1 in]
        n228 = Index Array(array=w367) -> (element=w366:cluster{string[]})  [unwired: 1 in]
        n229 = Unbundle(w371) -> ("Frame Rate"=w362:i32, "Compression"=w361:i32, "Size"=w364:u16)
        n230 = Unbundle(w366) -> (w365:string[])
        n231 = Index Array(array=w365, index=w364) -> (element=w363:string)
        n232 = Format Into String(format string="%s   %dfps   %d%%", w363, w362, w361) -> (resulting string=w368:string)  [unwired: 2 in, 1 out]
        n233 = Build Array(w368) -> (w369:string[])
        n234 = property on="DB Camera Config" class="Bool (strict)"("Strings [4]"=w369) -> ()  [unwired: 2 in, 2 out]
      }
      event "Motor.Enable": Value Change {
        n235 = event-data() -> ("NewVal"=w377:bool)  [unwired: 1 in]
        n236 = Unbundle("Motor") -> ("Value"=w376:dbl)  [unwired: 1 out]
        n237 = Select(t=w376, s=w377, f=0.0) -> (s? t:f=w374:dbl)
        n238 = call <vilib>:"NT Write Number.vi"("Numeric"=w374, "Name"=w373) -> ()  [unwired: 9 in, 1 out]
      }
      event "Test Slider": Value Change {
        n239 = event-data() -> ("NewVal"=w380:dbl)  [unwired: 1 in]
        n240 = call <vilib>:"NT Write Number.vi"("Numeric"=w380, "Name"=w381) -> ()  [unwired: 9 in, 1 out]
      }
      event "On/Off": Value Change {
        n241 = event-data() -> ("NewVal"=w385:bool)  [unwired: 1 in]
        n242 = Boolean To (0,1)(Boolean=w385) -> (0, 1=w384:i16)
        n243 = call <vilib>:"NT Write Number.vi"("Numeric"=w384, "Name"=w383) -> ()  [unwired: 9 in, 1 out]
      }
      event "Rev/Fwd": Value Change {
        n244 = event-data() -> ("NewVal.Forward"=w393:bool, "NewVal.Reverse"=w392:bool)  [unwired: 1 in]
        n245 = Boolean To (0,1)(Boolean=w393) -> (0, 1=w389:i16)
        n246 = Boolean To (0,1)(Boolean=w392) -> (0, 1=w391:i16)
        n247 = Negate(x=w391) -> (-x=w390:i16)
        n248 = Add(x=w389, y=w390) -> (x+y=w388:i16)
        n249 = call <vilib>:"NT Write Number.vi"("Numeric"=w388, "Name"=w387) -> ()  [unwired: 9 in, 1 out]
      }
      event "Test Ring": Value Change {
        n250 = event-data() -> ("NewVal"=w397:u16)  [unwired: 1 in]
        n251 = property on="Test Ring" class="Ring (strict)"() -> ("Strings []"=w398:string[])  [unwired: 2 in, 2 out]
        n252 = Index Array(array=w398, index=w397) -> (element=w396:string)
        n253 = call <vilib>:"NT Write String.vi"("String"=w396, "Name"=w395) -> ()  [unwired: 9 in, 1 out]
      }
      event "Rec Mode": Value Change {
        # "Update globals for recording mode and path to read log from.\nClear when logging and let NetworkTables set path for vision to\nuse."
        n254 = event-data() -> ("NewVal"=w408:enum32{"Stop", "Record", "Playback"})  [unwired: 1 in]
        n255 = global write "WPI_DashboardLogging Global.vi" "Logging Filename"(path "") -> ()
        n256 = global write "WPI_DashboardLogging Global.vi" "Recording"(w408) -> ()
        n257 = case shown="\"Stop\", \"Record\"" w408 {
          tunnel: w407 -> [_ w410 w418]
          tunnel: [_ _ w417] -> w404
          tunnel: [_ _ w416] -> _
          tunnel: w402 -> [_ _ w414]
          tunnel: cluster{i32, i32} {-250, 170} -> [_ _ w413]
          tunnel: [_ _ T14 {"Image Size"=TRUE, "Image Type"=TRUE, "Pixel Value"=TRUE, "ROI Information"=TRUE, "Zoom Factor"=FALSE} ("Image Information Shown:All Elements")] -> w400
          tunnel: [_ _ TRUE ("Zoom Factor")] -> w399
          frame Default {
          }
          frame "Stop", "Record" {
            # "Place Window too"
            n258 = invoke class="VI" method="FP.Close"(reference=w410) -> (reference out=w409:refnum<vi>)  [unwired: 2 in, 2 out]
            n259 = invoke class="VI" method="Abort VI"(reference=w409) -> ()  [unwired: 2 in, 3 out]
          }
          frame "Playback" {
            n260 = call "Open Playback Panel.vi"("Offset"=w413, "DB VI Ref"=w414, "Playback in"=w418) -> ("Playback out"=w415:refnum<vi>)  [unwired: 8 in]
            n261 = register-events(w415) -> (reference out=w417:refnum<event-registration>, error out=w416:errorcluster)  [unwired: 2 in]
          }
        }
        n262 = property on="Camera Image" class="ImageControl"("Image Information Shown"=w400, "Image Information Visible"=w399) -> ()  [unwired: 2 in, 2 out]
        n263 = call <vilib>:"WPI_DashboardNT Log FieldName Cache.vi"("Operation"=enum16{"Lookup/Add", "Index", "Clear"}."Clear") -> ()  [unwired: 8 in, 3 out]
      }
      event Panel Close {
        w419 = enum32{"Stop", "Record", "Playback"}."Stop" ("Rec Mode")
        n264 = event-data() -> ()  [unwired: 1 in, 4 out]
        n265 = local write "Rec Mode"(w419) -> ()
        n266 = global write "WPI_DashboardLogging Global.vi" "Recording"(w419) -> ()
      }
      event Panel Close {
        # "Abort playback window and ourself"
        n267 = event-data() -> ()  [unwired: 1 in, 4 out]
        n268 = invoke class="VI" method="FP.Close"(reference=w424) -> (reference out=w423:refnum<vi>)  [unwired: 2 in, 2 out]
        n269 = invoke class="VI" method="Abort VI"(reference=w423) -> (error out=w422:errorcluster)  [unwired: 2 in, 2 out]
        n270 = invoke class="VI" method="Abort VI"(error in=w422) -> ()  [unwired: 2 in, 3 out]
      }
    }
  }
  n271 = property on="On/Off" class="Bool (strict)"("Visible"=w25) -> ()  [unwired: 2 in, 2 out]
  n272 = property on="Motor" class="Clust (strict)"("Visible"=w25) -> ()  [unwired: 2 in, 2 out]
  n273 = property on="Progress" class="Clust (strict)"("Visible"=w25) -> ()  [unwired: 2 in, 2 out]
  n274 = property on="Test Ring" class="Ring (strict)"("Visible"=w25) -> ()  [unwired: 2 in, 2 out]
  n275 = property on="Rev/Fwd" class="Clust (strict)"("Visible"=w25) -> ()  [unwired: 2 in, 2 out]
  n276 = local write "DB Camera Config"(w25) -> ()
  n277 = property on="Camera Settings" class="Clust (strict)"("Visible"=w25) -> ()  [unwired: 2 in, 2 out]
  n278 = global write "WPI_DashboardLogging Global.vi" "Recording"(w8) -> ()
  n279 = local write "Rec Mode"(w8) -> ()
